vi "BRig_dataLC_Wrong_Trial_l1.vi"() -> (2 "output_Wrong_Trial":i32)   [LabVIEW 2014]
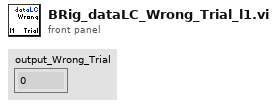
[diagram p1: front panel]
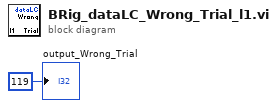
[diagram p0: block diagram]
diagram:
  "output_Wrong_Trial" <- 119 ("output_iBlock")
